vi "Newly Updated Micronix Approach.vi"() -> ()   [LabVIEW 2022 SP3]
uses:
  <vilib>/DAQmx/read.llb/DAQmx Read (Counter U32 1Chan 1Samp).vi
  <vilib>/DAQmx/miscellaneous.llb/DAQmx Fill In Error Info.vi
  <resource>/objmgr/daqmx.rc
  <vilib>/DAQmx/create/channels.llb/DAQmx Create Channel (CI-Count Edges).vi
panel:
  in  "Retract 5 um":bool
  in  "Retract 1mm":bool
  in  "Trigger Edge":i32(ring)=10171 items=["Rising"=10280, "Falling"=10171]
  in  "Trigger Terminal":tag="/Dev1/PFI1"
  in  "physical channels":tag
  in  "Controller #":string
  in  "Polarity":bool caption="pos      neg"
  in  "Counter":u32
  in  "End Approach":bool
  in  "Start Approach":bool
  in  "Stop":bool
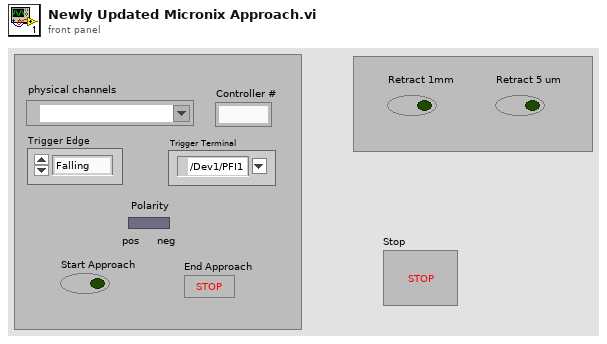
[diagram p1: front panel]
types:
  T1 = cluster{"P type":u16, "VISA resource name out":refnum<visa-resource-name>, " Terminator":string, "Timeout":i32}
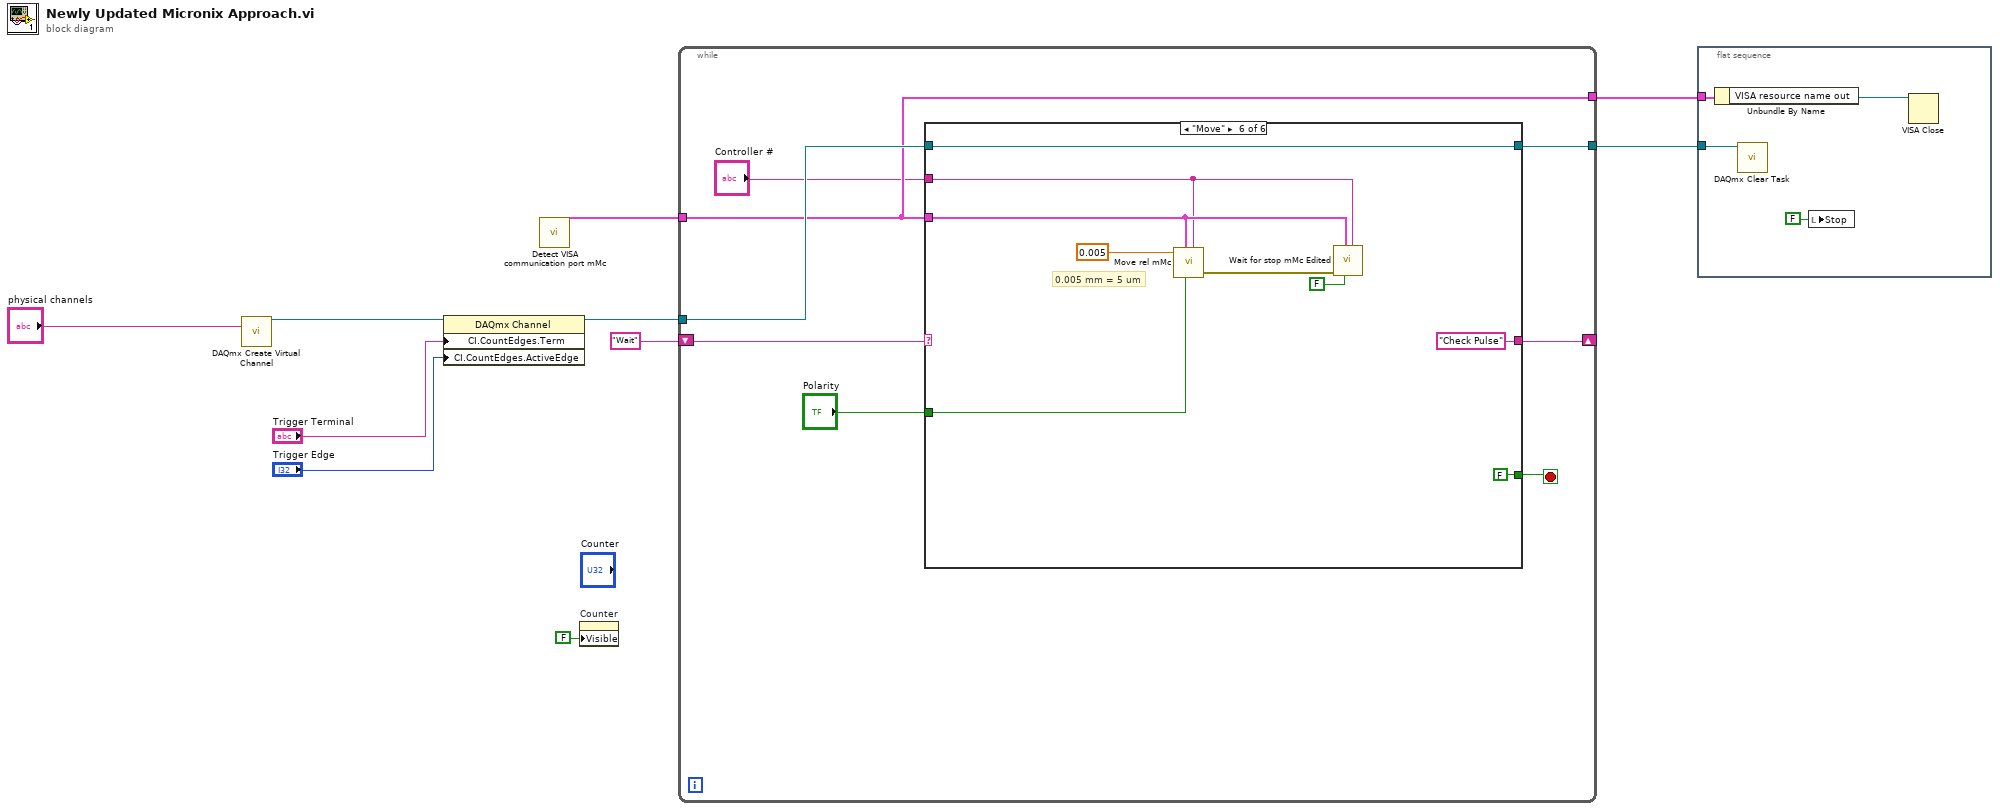
[diagram p0: block diagram]
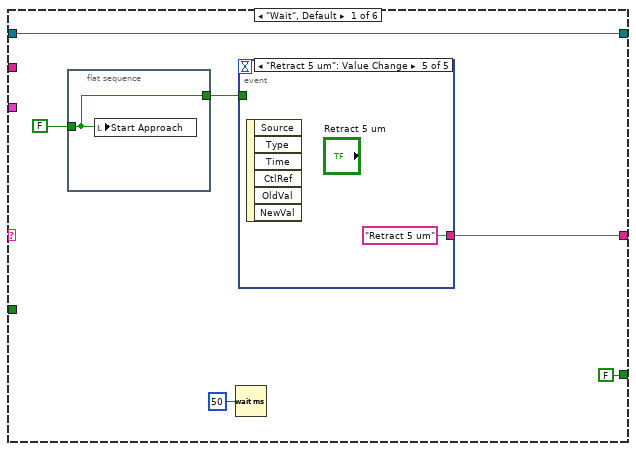
[diagram p2: hidden frame]
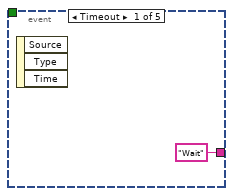
[diagram p3: hidden frame]
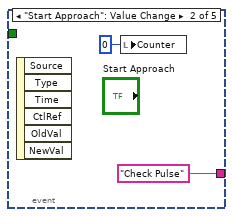
[diagram p4: hidden frame]
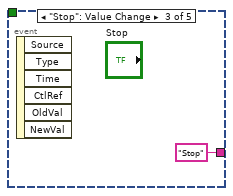
[diagram p5: hidden frame]
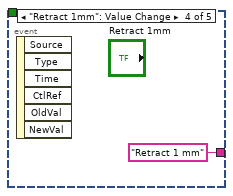
[diagram p6: hidden frame]
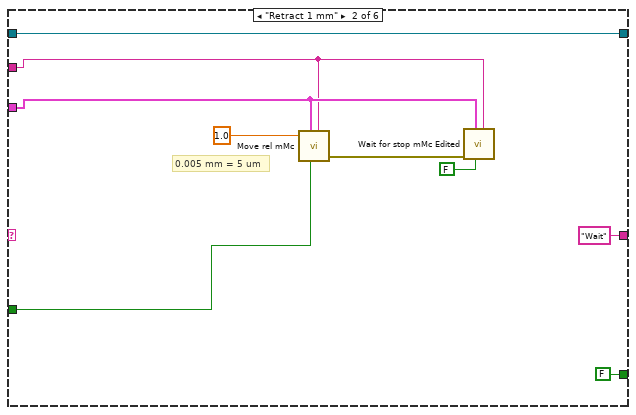
[diagram p7: hidden frame]
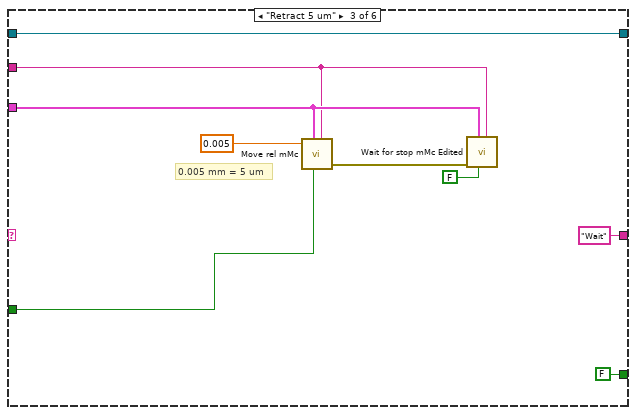
[diagram p8: hidden frame]
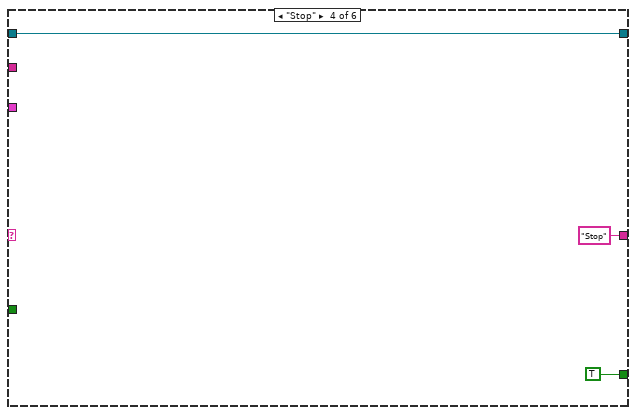
[diagram p9: hidden frame]
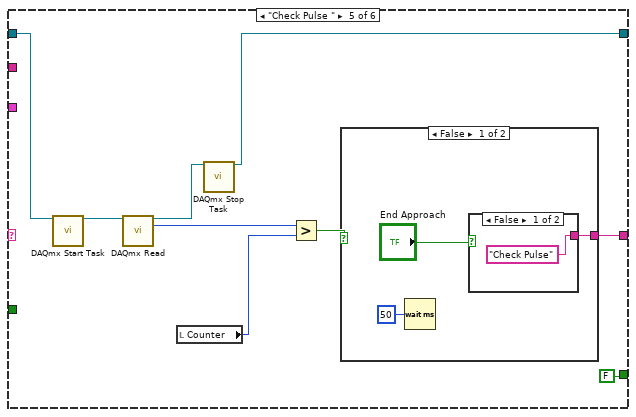
[diagram p10: hidden frame]
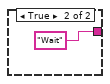
[diagram p11: hidden frame]
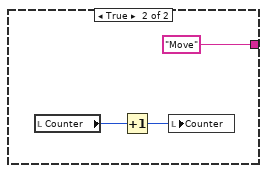
[diagram p12: hidden frame]
diagram:
  n1 = call-poly <vilib>:"DAQmx Create Virtual Channel.vi"("counter"="physical channels") -> ("task out"=w5:refnum<k21>)  [unwired: 13 in, 1 out]
  n2 = property class="DAQmx Channel"(reference=w5, "CI.CountEdges.Term"="Trigger Terminal", "CI.CountEdges.ActiveEdge"="Trigger Edge") -> (reference out=w4:refnum<k21>)  [unwired: 1 in, 1 out]
  n3 = call "Detect VISA communication port mMc.vi"() -> ("Port"=w9:T1)  [unwired: 6 in, 3 out]
  n4 = property on="Counter" class="DigNum (strict)"("Visible"=FALSE) -> ()  [unwired: 2 in, 2 out]
  n5 = while {
    shift-right: [w18] -> _
    shift-left: "Wait" -> [w17]
    tunnel: w9 -> [w13]
    tunnel: w4 -> [w16]
    tunnel: [w15] -> w2
    tunnel: [w13] -> w1
    stop <- w14 stop-if-true
    n6 = case shown="\"Move\"" w17 {
      tunnel: [w24 "Wait" "Wait" "Stop" w59 "Check Pulse"] -> w18
      tunnel: w13 -> [_ w34 w42 _ _ w74]
      tunnel: w16 -> [w22 w40 w47 w51 w57 w73]
      tunnel: [w22 w40 w47 w51 w54 w73] -> w15
      tunnel: [FALSE FALSE FALSE TRUE FALSE FALSE] -> w14
      tunnel: "Controller #" -> [_ w33 w41 _ _ w71]
      tunnel: "Polarity" -> [_ w32 w43 _ _ w70]
      frame "Wait", Default {
        n7 = flat-sequence {
          tunnel: FALSE -> [w25]
          tunnel: [w25] -> w20
          frame #0 {
            n8 = local write "Start Approach"(w25) -> ()
          }
        }
        n9 = Wait (ms)(milliseconds to wait=u32 50) -> ()  [unwired: 1 out]
        n10 = event shown="[4] \"Retract 5 um\": Value Change" {
          selector: _ -> [_ _ _ _ _]
          dyn-events: _ -> [_ _ _ _ _]
          timeout: _ -> [_ _ _ _ _]
          tunnel: ["Wait" "Check Pulse" "Stop" "Retract 1 mm" "Retract 5 um"] -> w24
          tunnel: w20 -> [_ _ _ _ _]
          event Timeout {
            n11 = event-data() -> ()  [unwired: 1 in, 3 out]
          }
          event "Start Approach": Value Change {
            n12 = event-data() -> ()  [unwired: 1 in, 6 out]
            n13 = local write "Counter"(u32 0 ("Counter")) -> ()
          }
          event "Stop": Value Change {
            n14 = event-data() -> ()  [unwired: 1 in, 6 out]
          }
          event "Retract 1mm": Value Change {
            n15 = event-data() -> ()  [unwired: 1 in, 6 out]
          }
          event "Retract 5 um": Value Change {
            n16 = event-data() -> ()  [unwired: 1 in, 6 out]
          }
        }
      }
      frame "Retract 1 mm" {
        # "0.005 mm = 5 um"
        n17 = call "Move rel mMc.vi"("position incr"=1.0, "Port"=w34, "rev dir?"=w32, "Controller #"=w33) -> ("error out"=w37:errorcluster)  [unwired: 5 in]
        n18 = call "Wait for stop mMc Edited.vi"("Controller #"=w33, "wait for in pos"=FALSE, "Port"=w34, "error in (no error)"=w37) -> ()  [unwired: 7 in, 1 out]
      }
      frame "Retract 5 um" {
        # "0.005 mm = 5 um"
        n19 = call "Move rel mMc.vi"("position incr"=0.005, "Port"=w42, "rev dir?"=w43, "Controller #"=w41) -> ("error out"=w46:errorcluster)  [unwired: 5 in]
        n20 = call "Wait for stop mMc Edited.vi"("Controller #"=w41, "wait for in pos"=FALSE, "Port"=w42, "error in (no error)"=w46) -> ()  [unwired: 7 in, 1 out]
      }
      frame "Stop" {
      }
      frame "Check Pulse " {
        n21 = call <vilib>:"DAQmx Start Task.vi"("task/channels in"=w57) -> ("task out"=w56:refnum<k21>)  [unwired: 13 in, 1 out]
        n22 = call-poly <vilib>:"DAQmx Read.vi"("task/channels in"=w56) -> ("task out"=w55:refnum<k21>, "data"=w60:u32)  [unwired: 12 in, 1 out]
        n23 = local read "Counter"() -> (w58:u32)
        n24 = call <vilib>:"DAQmx Stop Task.vi"("task/channels in"=w55) -> ("task out"=w54:refnum<k21>)  [unwired: 13 in, 1 out]
        n25 = Greater?(x=w60, y=w58) -> (0:w61:bool)
        n26 = case shown="False" w61 {
          tunnel: [w63 "Move"] -> w59
          frame False {
            n27 = Wait (ms)(milliseconds to wait=u32 50) -> ()  [unwired: 1 out]
            n28 = case shown="False" "End Approach" {
              tunnel: ["Check Pulse" "Wait"] -> w63
              frame False {
              }
              frame True {
              }
            }
          }
          frame True {
            n29 = local read "Counter"() -> (w68:u32)
            n30 = Increment(x=w68) -> (x+1=w67:u32)
            n31 = local write "Counter"(w67) -> ()
          }
        }
      }
      frame "Move" {
        # "0.005 mm = 5 um"
        n32 = call "Move rel mMc.vi"("position incr"=0.005, "Port"=w74, "rev dir?"=w70, "Controller #"=w71) -> ("error out"=w77:errorcluster)  [unwired: 5 in]
        n33 = call "Wait for stop mMc Edited.vi"("Controller #"=w71, "wait for in pos"=FALSE, "Port"=w74, "error in (no error)"=w77) -> ()  [unwired: 7 in, 1 out]
      }
    }
  }
  n34 = flat-sequence {
    tunnel: w1 -> [w79]
    tunnel: w2 -> [w80]
    frame #0 {
      n35 = Unbundle By Name(w79) -> ("VISA resource name out"=w82:refnum<visa-resource-name>)
      n36 = call <vilib>:"DAQmx Clear Task.vi"("task in"=w80) -> ()  [unwired: 14 in, 1 out]
      n37 = local write "Stop"(FALSE ("Stop")) -> ()
      n38 = VISA Close(VISA resource name=w82) -> ()  [unwired: 1 in, 1 out]
    }
  }
